vi "New SenseHat.Display.vi"(8 "error in (no error)":errorcluster, 11 "MainI2CDevice":refnum<class "mainI2CDevice.lvclass">) -> (0 "error out":errorcluster, 3 "senseHatDisplay out":refnum<class "RPI.SenseHat.Display.lvclass">)   [LabVIEW 2020, in "RPI.SenseHat.Display.lvlib" / "RPI.SenseHat.Display.lvclass"]
doc: "Instantiates a RPI.SenseHat.Display object.\n\nNote: opens the I2C communication."
uses:
  RPI.SenseHat.Display.lvclass
  RPI/Classes/mainI2CDevice/mainI2CDevice.lvclass
  TypeDefs/Display Direction.ctl
  RPI.SenseHat.Display.lvclass/RPI.SenseHat.Display.ctl
  RPI.SenseHat.Display.lvlib
  Image/Image.lvclass
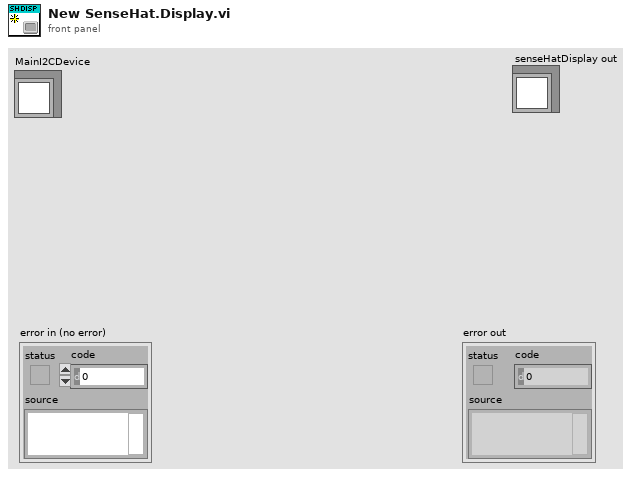
[diagram p1: front panel]
types:
  T1 = typedef "RPI.SenseHat.Display.lvlib/Display Direction.ctl" = enum16{"deg0", "deg90", "deg180", "deg270"}
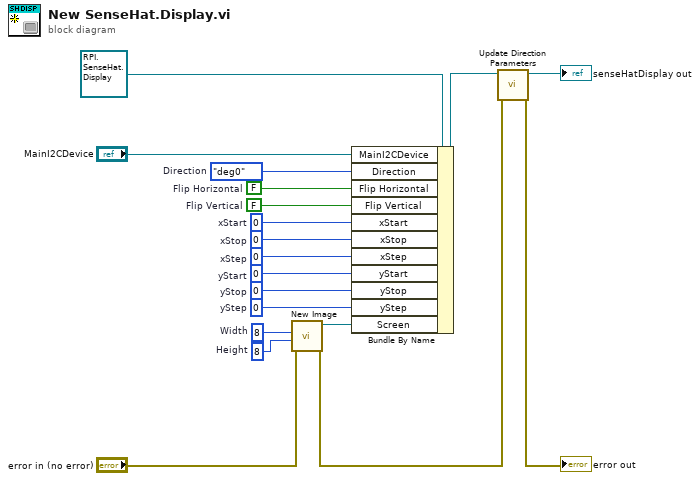
[diagram p0: block diagram]
diagram:
  w5 = 8  # Width
  w6 = 8  # Height
  w8 = 0  # yStep
  w9 = 0  # yStop
  w10 = 0  # yStart
  w11 = 0  # xStep
  w12 = 0  # xStop
  w13 = 0  # xStart
  w14 = FALSE  # Flip Vertical
  w15 = FALSE  # Flip Horizontal
  w16 = Display_Direction."deg0"  # Direction
  n1 = call "New Image.vi"("error in (no error)"="error in (no error)", "Height"=w6, "Width"=w5) -> ("error out"=w3:errorcluster, "Image out"=w7:refnum<class "Image.lvclass">)  [unwired: 7 in]
  n2 = Bundle By Name(cluster=refnum<class "RPI.SenseHat.Display.lvclass"> refnum ("senseHatDisplay in"), "MainI2CDevice"="MainI2CDevice", "Direction"=w16, "Flip Horizontal"=w15, "Flip Vertical"=w14, "xStart"=w13, "xStop"=w12, "xStep"=w11, "yStart"=w10, "yStop"=w9, "yStep"=w8, "Screen"=w7) -> (w17:refnum<class "RPI.SenseHat.Display.lvclass">)
  n3 = call "Update Direction Parameters.vi"("error in (no error)"=w3, "senseHatDisplay in"=w17) -> ("error out"=→"error out":errorcluster, "senseHatDisplay out"=→"senseHatDisplay out":refnum<class "RPI.SenseHat.Display.lvclass">)  [unwired: 8 in]
